vi "SU_Set.vi"(6 "Direction":T1 items=["Positive", "Negative"], 8 "error in (no error)":errorcluster, 9 "Step Amplitude":i32, 10 "Axis Number":i32, 11 "Agilis in":T2) -> (0 "error out":errorcluster, 3 "Agilis out":T2)   [LabVIEW 2016, in "Drivers.lvlib" / "Agilis.lvlib"]
doc: "Returns the step amplitude setting in either positive or negative direction."
uses:
  Agilis.lvlib
  AgilisCmdLib Refnum.ctl
  D:/Trace Grabber/Drivers/Agilis/AgilisCmdLib.dll
  AgilisCmdLib.dll
  Direction.ctl
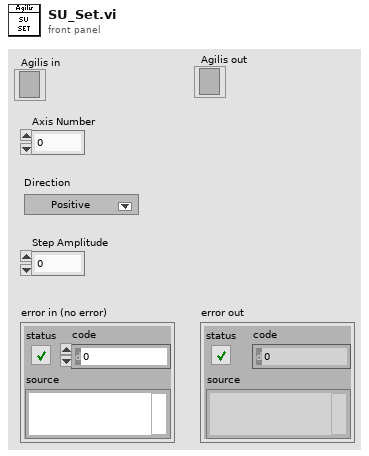
[diagram p1: front panel]
types:
  T1 = typedef "Drivers.lvlib/Agilis.lvlib/Direction.ctl" = u8
  T2 = typedef "Drivers.lvlib/Agilis.lvlib/AgilisCmdLib Refnum.ctl" = refnum<k24>
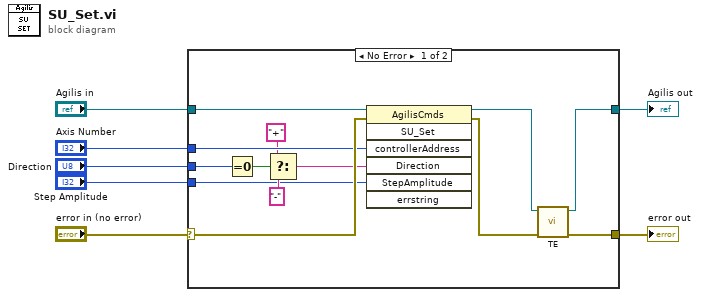
[diagram p0: block diagram]
diagram:
  n1 = case shown="No Error" "error in (no error)" {
    selector: "error in (no error)" -> [w19 w22]
    tunnel: "Agilis in" -> [w20 w21]
    tunnel: [w8 w21] -> w5
    tunnel: [w10 w22] -> w4
    tunnel: "Axis Number" -> [w18 _]
    tunnel: "Direction" -> [w17 _]
    tunnel: "Step Amplitude" -> [w12 _]
    frame No Error {
      n2 = Equal To 0?(x=w17) -> (x = 0?=w16:bool)
      n3 = Select(t="+" ("Direction"), s=w16, f="-" ("Direction")) -> (s? t:f=w14:string)
      n4 = invoke class="AgilisCmds" method="SU_Set"(reference=w20, error in=w19, "controllerAddress"=w18, "Direction"=w14, "StepAmplitude"=w12) -> (reference out=w9:T2, error out=w11:errorcluster)  [unwired: 2 in, 5 out]
      n5 = call "TE.vi"("error in (no error)"=w11, "Agilis in"=w9) -> ("error out"=w10:errorcluster, "Agilis out"=w8:T2)  [unwired: 8 in]
    }
    frame Error {
    }
  }
  "Agilis out" <- w5
  "error out" <- w4
